vi "Write Disabled Items.vi"(5 "Disabled Items":i32[](array[numeric]), 9 "NamedNumeric in":refnum<class "NamedNumeric.lvclass">) -> (3 "NamedNumeric out":refnum<class "NamedNumeric.lvclass">)   [LabVIEW 2014, in "NamedNumeric.lvclass"]
uses:
  NamedNumeric.lvclass
  NamedNumeric.lvclass/NamedNumeric.ctl
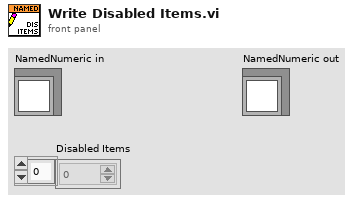
[diagram p1: front panel]
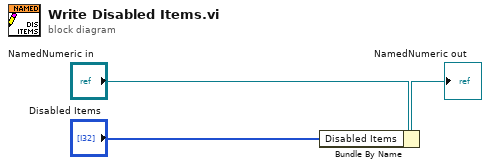
[diagram p0: block diagram]
diagram:
  n1 = Bundle By Name(cluster="NamedNumeric in", "Disabled Items"="Disabled Items") -> (→"NamedNumeric out":refnum<class "NamedNumeric.lvclass">)
